vi "2 TuningConstants.vi"() -> ()   [LabVIEW 2011]
uses:
  2 Typedefs/PI Constants.ctl
  2 Typedefs/Goodness Weightings.ctl
  2 Typedefs/Apparent Wind Mode.ctl
  0x2-OCU-Think Comm/0x2 Typedefs/Sail Setting Tuning.ctl
panel:
  in  "Aggressiveness":dbl
  in  "Irons Range":dbl=40.0 step=0.1
  in  "Sail Setting Options":T1={"Linear\nMode"=FALSE, "Sails Full In Point"=45.0, "Sails Full Out Point"=180.0} {"Sails Full Out Point" step=0.1; "Sails Full In Point" step=0.1}
  in  "Apparent Wind Mode":T2 {"Desired Apparent\nWind Direction" step=0.1}
  in  "Waypoint Tuning Constant":dbl=80.0 step=0.1
  in  "Wind Adjustment":dbl=0.2 step=0.1
  in  "Goodness Weightings":T3={"Target Importance"=0.98, "No Sail Importance"=1.0, "Change Importance"=0.2, "Pure Waypoint \nImportance"=0.0, "Pure Wind \nImportance"=0.0} {"Pure Wind \nImportance" min=0.0 step=0.2; "Pure Waypoint \nImportance" min=0.0 step=0.2; "Change Importance" min=0.0 step=0.2; "No Sail Importance" min=0.0 step=0.2; "Target Importance" min=0.0 step=0.2}
  in  "No Sail Tuning Quotient":dbl=0.05 step=0.1
  in  "PI Constants":T4={"Proportional Gain"=1.0, "Integral Time"=0.0, "Derivative Time"=0.0}
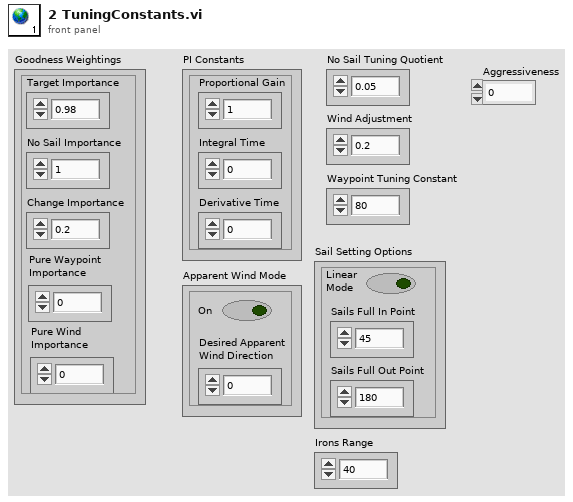
[diagram p1: front panel]
types:
  T1 = typedef "Sail Setting Tuning.ctl" = cluster{"Linear\nMode":bool, "Sails Full In Point":dbl, "Sails Full Out Point":dbl}
  T2 = typedef "Apparent Wind Mode.ctl" = cluster{"Desired Apparent\nWind Direction":dbl, "On":bool}
  T3 = typedef "Goodness Weightings.ctl" = cluster{"Target Importance":dbl, "No Sail Importance":dbl, "Change Importance":dbl, "Pure Waypoint \nImportance":dbl, "Pure Wind \nImportance":dbl}
  T4 = typedef "PI Constants.ctl" = cluster{"Proportional Gain":dbl, "Integral Time":dbl, "Derivative Time":dbl}
diagram:
